vi "UtilityLib.get help text.vi"(1 "helpType":T1, 2 "VIDescription":string) -> (0 "helpText":string)   [LabVIEW 2015, in "UtilityLib.lvlib"]
doc: "Gets the help text on a specific subject like \"help on menus...\"), by looking for text that is surrounded by a specific keyword. The keywords have the following format.\n\nSUBJECTHelpStart\nblabla\nSUBJECTHelpStop\n\nThe keyword SUBJECT may have the following values\nmenu: to be used, to obtain help on the menus and options\ndescription: to be used, to obtain a description of the program\nspecial0: user specific\nspecial1: user specific\nspecial2: user specific\n\nThere exist also two other help types:\nunknown: returns the full description of the calling VI\nabout: returns the full description of the owning library of the calling VI"
uses:
  UtilityLib.lvlib
  UtilityLib.helpType.ctl
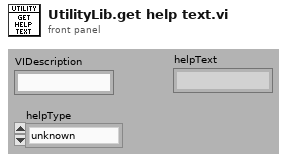
[diagram p1: front panel]
types:
  T1 = typedef "UtilityLib.lvlib/UtilityLib.helpType.ctl" = enum16{"unknown", "menu", "description", "about", "special0", "special1", "special2"}
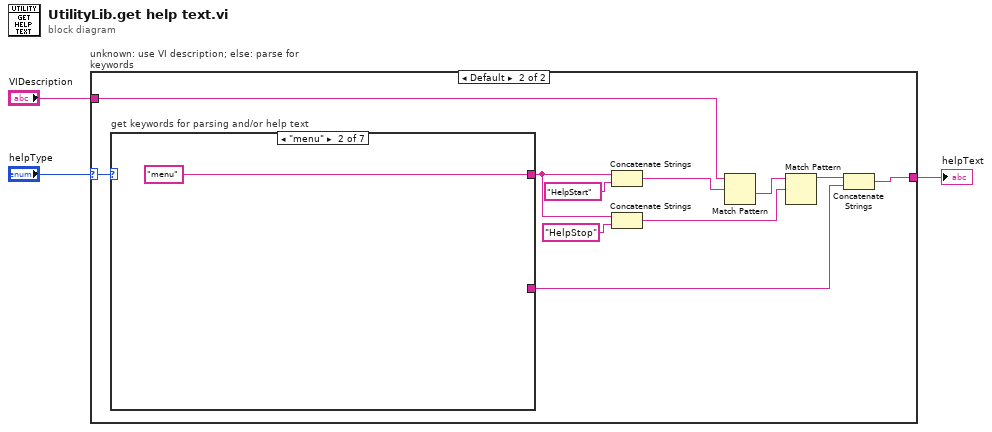
[diagram p0: block diagram]
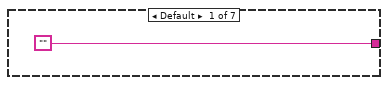
[diagram p3: hidden frame]
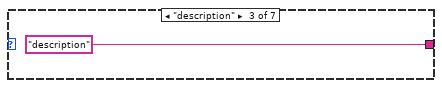
[diagram p4: hidden frame]
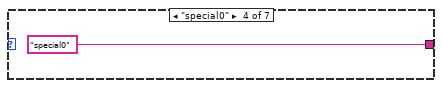
[diagram p5: hidden frame]
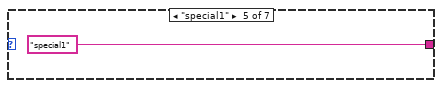
[diagram p6: hidden frame]
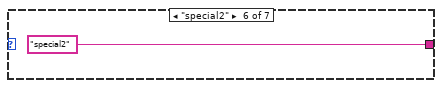
[diagram p7: hidden frame]
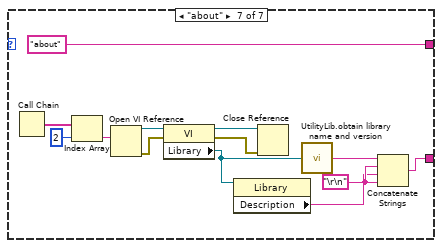
[diagram p8: hidden frame]
diagram:
  n1 = case "unknown: use VI description; else: parse for keywords" shown="Default" "helpType" {
    selector: "helpType" -> [_ w7]
    tunnel: [w4 w6] -> w3
    tunnel: "VIDescription" -> [w4 w14]
    frame "unknown" {
    }
    frame Default {
      n2 = case "get keywords for parsing and/or help text" shown="\"menu\"" w7 {
        tunnel: ["" ("Empty String Constant") "menu" "description" "special0" "special1" "special2" "about"] -> w9
        tunnel: [_ _ _ _ _ _ w25] -> w5
        frame Default {
        }
        frame "menu" {
        }
        frame "description" {
        }
        frame "special0" {
        }
        frame "special1" {
        }
        frame "special2" {
        }
        frame "about" {
          w23 = "\r\n"
          n3 = Call Chain() -> (call chain=w33:string[])
          n4 = Index Array(array=w33, index=2) -> (element=w31:string)
          n5 = Open VI Reference(vi path=w31) -> (vi reference=w29:refnum<vi>, error out=w30:errorcluster)  [unwired: 5 in]
          n6 = property class="VI"(reference=w29, error in=w30) -> (reference out=w27:refnum<vi>, error out=w28:errorcluster, "Library"=w24:refnum<vi>)
          n7 = property class="Library"(reference=w24) -> ("Description"=w22:string)  [unwired: 1 in, 2 out]
          n8 = Close Reference(reference=w27, error in (no error)=w28) -> ()  [unwired: 1 out]
          n9 = call "UtilityLib.obtain library name and version.vi"("Library"=w24) -> ("nameAndVersion"=w26:string)
          n10 = Concatenate Strings(w26, w23, w22, w23) -> (w25:string)
        }
      }
      n11 = Concatenate Strings(w9, "HelpStart" ("string")) -> (w13:string)
      n12 = Concatenate Strings(w9, "HelpStop" ("string")) -> (w12:string)
      n13 = Match Pattern(string=w14, regular expression=w13) -> (after substring=w11:string)  [unwired: 1 in, 3 out]
      n14 = Match Pattern(string=w11, regular expression=w12) -> (before substring=w15:string)  [unwired: 1 in, 3 out]
      n15 = Concatenate Strings(w15, w5) -> (w6:string)
    }
  }
  "helpText" <- w3
